vi "update_lights.vi"(9 "Lights":T1, 10 "Lighting Properties":T2, 11 "Scene:New Object":refnum<vi>) -> (3 "Scene:New Object 2":refnum<vi>)   [LabVIEW 2020, in "3DPC_SurfacePlot.xctl"]
uses:
  <vilib>/Native 3D Graph/xcontrol/3DPC_SurfacePlot.xctl
  <vilib>/Native 3D Graph/typedefs/prop_lighting.ctl
  <vilib>/Native 3D Graph/typedefs/prop_lights.ctl
  <vilib>/picture/3D Picture Control/NI_3D Picture Control.lvlib
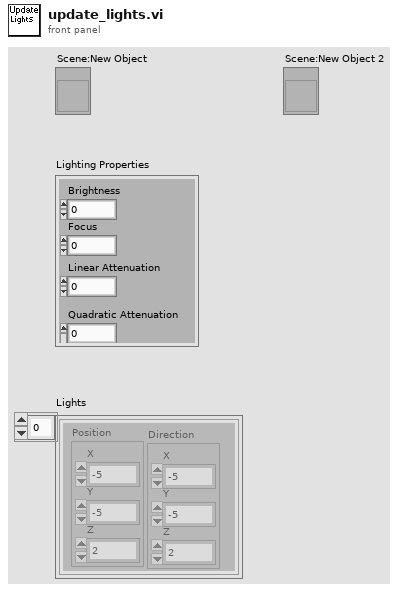
[diagram p1: front panel]
types:
  T1 = typedef "3DPC_SurfacePlot.xctl/prop_lights.ctl" = cluster{"Position":cluster{"X":sgl, "Y":sgl, "Z":sgl}, "Direction":cluster{"X":sgl, "Y":sgl, "Z":sgl}}[]
  T2 = typedef "3DPC_SurfacePlot.xctl/prop_lighting.ctl" = cluster{"Brightness":i32, "Focus":dbl, "Linear Attenuation":dbl, "Quadratic Attenuation":dbl}
  T3 = typedef "LVAttenuationTypeDef.ctl" = cluster{"Constant":sgl, "Linear":sgl, "Quadratic":sgl}
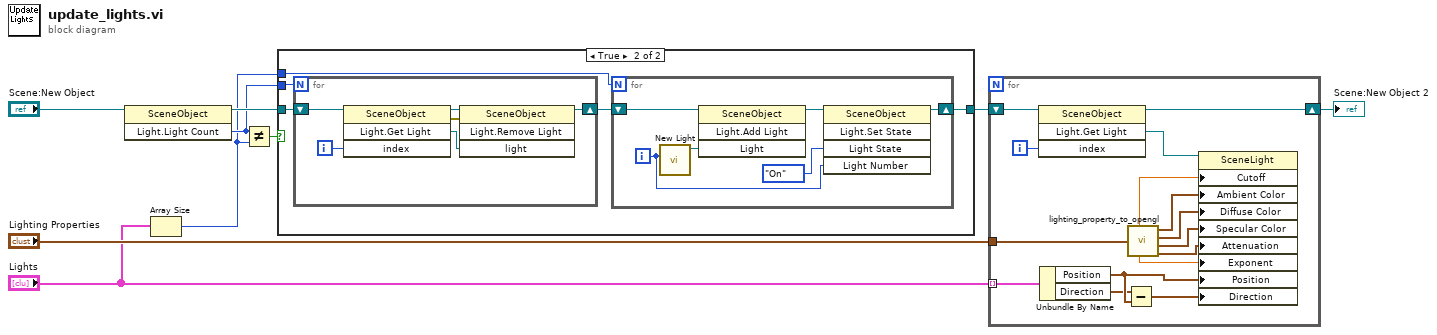
[diagram p0: block diagram]
diagram:
  n1 = invoke class="SceneObject" method="Light.Light Count"(reference="Scene:New Object") -> (reference out=w6:refnum<vi>, "Light Count"=w4:i32)  [unwired: 2 in, 1 out]
  n2 = Array Size(array="Lights") -> (size(s)=w1:i32)
  n3 = Not Equal?(x=w4, y=w1) -> (x != y?=w2:bool)
  n4 = case shown="True" w2 {
    tunnel: w6 -> [w10 w15]
    tunnel: [w10 w12] -> w5
    tunnel: w4 -> [_ w14]
    tunnel: w1 -> [_ w11]
    frame False {
    }
    frame True {
      n5 = for {
        N: w14 -> [_]
        shift-right: [w22] -> w13
        shift-left: w15 -> [w23]
        i -> [w24]
        n6 = invoke class="SceneObject" method="Light.Get Light"(reference=w23, "index"=w24) -> (reference out=w27:refnum<vi>, error out=w26:errorcluster, "Get Light"=w25:refnum<vi>)  [unwired: 2 in, 1 out]
        n7 = invoke class="SceneObject" method="Light.Remove Light"(reference=w27, error in=w26, "light"=w25) -> (reference out=w22:refnum<vi>)  [unwired: 1 in, 3 out]
      }
      n8 = for {
        N: w11 -> [_]
        shift-right: [w19] -> w12
        shift-left: w13 -> [w18]
        i -> [w17]
        n9 = call <vilib>:"New Light.vi"("Light Number"=w17) -> ("New Light Refnum"=w21:refnum<vi>)  [unwired: 2 in, 8 out]
        n10 = invoke class="SceneObject" method="Light.Add Light"(reference=w18, "Light"=w21) -> (reference out=w20:refnum<vi>)  [unwired: 2 in, 3 out]
        n11 = invoke class="SceneObject" method="Light.Set State"(reference=w20, "Light State"=enum16{"Inherit Value", "Off", "On"}."On", "Light Number"=w17) -> (reference out=w19:refnum<vi>)  [unwired: 2 in, 4 out]
      }
    }
  }
  n12 = for {
    tunnel: "Lighting Properties" -> [w42]
    tunnel: "Lights" -> [w35] mode=indexing
    shift-right: [w29] -> w8
    shift-left: w5 -> [w30]
    i -> [w31]
    n13 = invoke class="SceneObject" method="Light.Get Light"(reference=w30, "index"=w31) -> (reference out=w29:refnum<vi>, "Get Light"=w28:refnum<vi>)  [unwired: 2 in, 2 out]
    n14 = Unbundle By Name(w35) -> ("Position"=w34:cluster{"X":sgl, "Y":sgl, "Z":sgl}, "Direction"=w33:cluster{"X":sgl, "Y":sgl, "Z":sgl})
    n15 = Subtract(x=w33, y=w34) -> (x-y=w32:cluster{"X":sgl, "Y":sgl, "Z":sgl})
    n16 = call <vilib>:"lighting_property_to_opengl.vi"("Lighting Properties"=w42) -> ("Cutoff"=w41:dbl, "Exponent"=w36:dbl, "Ambient Color"=w40:cluster{"R":sgl, "G":sgl, "B":sgl, "A":sgl}, "Diffuse Color"=w39:cluster{"R":sgl, "G":sgl, "B":sgl, "A":sgl}, "Specular Color"=w38:cluster{"R":sgl, "G":sgl, "B":sgl, "A":sgl}, "Attenuation"=w37:T3)  [unwired: 2 out]
    n17 = property class="SceneLight"(reference=w28, "Cutoff"=w41, "Ambient Color"=w40, "Diffuse Color"=w39, "Specular Color"=w38, "Attenuation"=w37, "Exponent"=w36, "Position"=w34, "Direction"=w32) -> ()  [unwired: 1 in, 2 out]
  }
  "Scene:New Object 2" <- w8
